vi "CODMn断电保存全局变量.vi"() -> ()   [LabVIEW 2016, in "斯坦道CODMn.lvlib"]
panel:
  in  "远程校准量程":enum16{"L", "H"}(ring)
  in  "远程自动校准浓度":dbl
  in  "CODMn仪器参数":T1 {"单位" items=["ug/L", "mg/L"]}
  out "测量数据区":T2 {"单位" items=["ug/L", "mg/L", "ppm", "mg/m3", "cm", "ppb", "ug/m3", "%", "nmol/mol", "umol/mol", "MPN/L", "MPN/100ml", "ng/m3", "NTU", "无量纲", "ms/cm", "us/cm", "℃", "mV", "万个/L"]}
  in  "运行周期":T3={"运行模式"=enum."维护模式", "质控频次"=enum."关闭", "空白核查时间"=2, "跨度核查时间"=6, "24H周期设置"=[]} {"跨度核查时间" items=["00H", "01H", "02H", "03H", "04H", "05H", "06H", "07H", "08H", "09H", "10H", "11H", "12H", "13H", "14H", "15H", "16H", "17H", "18H", "19H", "20H", "21H", "22H", "23H", "关闭"]; "空白核查时间" items=["00H", "01H", "02H", "03H", "04H", "05H", "06H", "07H", "08H", "09H", "10H", "11H", "12H", "13H", "14H", "15H", "16H", "17H", "18H", "19H", "20H", "21H", "22H", "23H", "关闭"]}
  in  "标样核查量程选择":enum32{"H", "L", "AUTO"}(ring)=enum."AUTO"
  in  "标样浓度":dbl
  in  "零点核查量程选择":enum32{"H", "L", "AUTO"}(ring)=enum."AUTO"
  in  "零点核查浓度":dbl
  in  "MB通信方式选择":enum16{"串口", "TCP"}(ring)
  in  "PORT":string="502"
  in  "IP":string="192.168.1.202"
  in  "Slave ID":u8=1
  in  "Serial Config":T4={"baud rate (bps)"=115200, "stop bits"=10, "parity"=0, "flow control"=0, "timeout"=1000, "retries"=1} {"stop bits" items=["1.0"=10, "1.5"=15, "2.0"=20]; "flow control" items=["None", "XON/XOFF", "RTS/CTS", "XON/XOFF & RTS/CTS", "DTR/DSR", "XON/XOFF & DTR/DSR"]; "parity" items=["None", "Odd", "Even", "Mark", "Space"]}
  in  "Error in":errorcluster
  in  "VISA resource name":refnum<visa-resource-name>="COM4" caption="VISA资源名称"
  in  "常规版/认证版":enum16{"常规版", "认证版", "浮台版"}(ring)
  out "启动时间":timestamp format="%<%Y/%m/%d %H:%M:%S>T"
  in  "高切低阈值:":dbl
  in  "低切高阈值:":dbl
  in  "自动切换量程:":enum16{"关闭", "自动切换测一次", "自动切换测两次"}(ring)
  in  "跨度液浓度":dbl
  in  "CODMn跨度量程选择":enum32{"H", "L", "AUTO"}(ring)=enum."AUTO"
  out "测量模式(公式)":u16(ring) items=["水样测试"=1, "标样核查"=2, "零点核查"=3, "跨度核查"=4, "空白测试"=5, "平行样"=6, "加标回收"=7]
  in  "定时控制":T5
  # "标样浓度："
  # "跨度液浓度："
  # "标样量程选择："
  # "零点核查浓度："
  # "零点量程选择："
  # "MBTCP参数"
  # "mg/L"
  # "运行模式："
  # "质控频次："
  # "空白核查时间："
  # "跨度核查时间："
  # "MB串口参数"
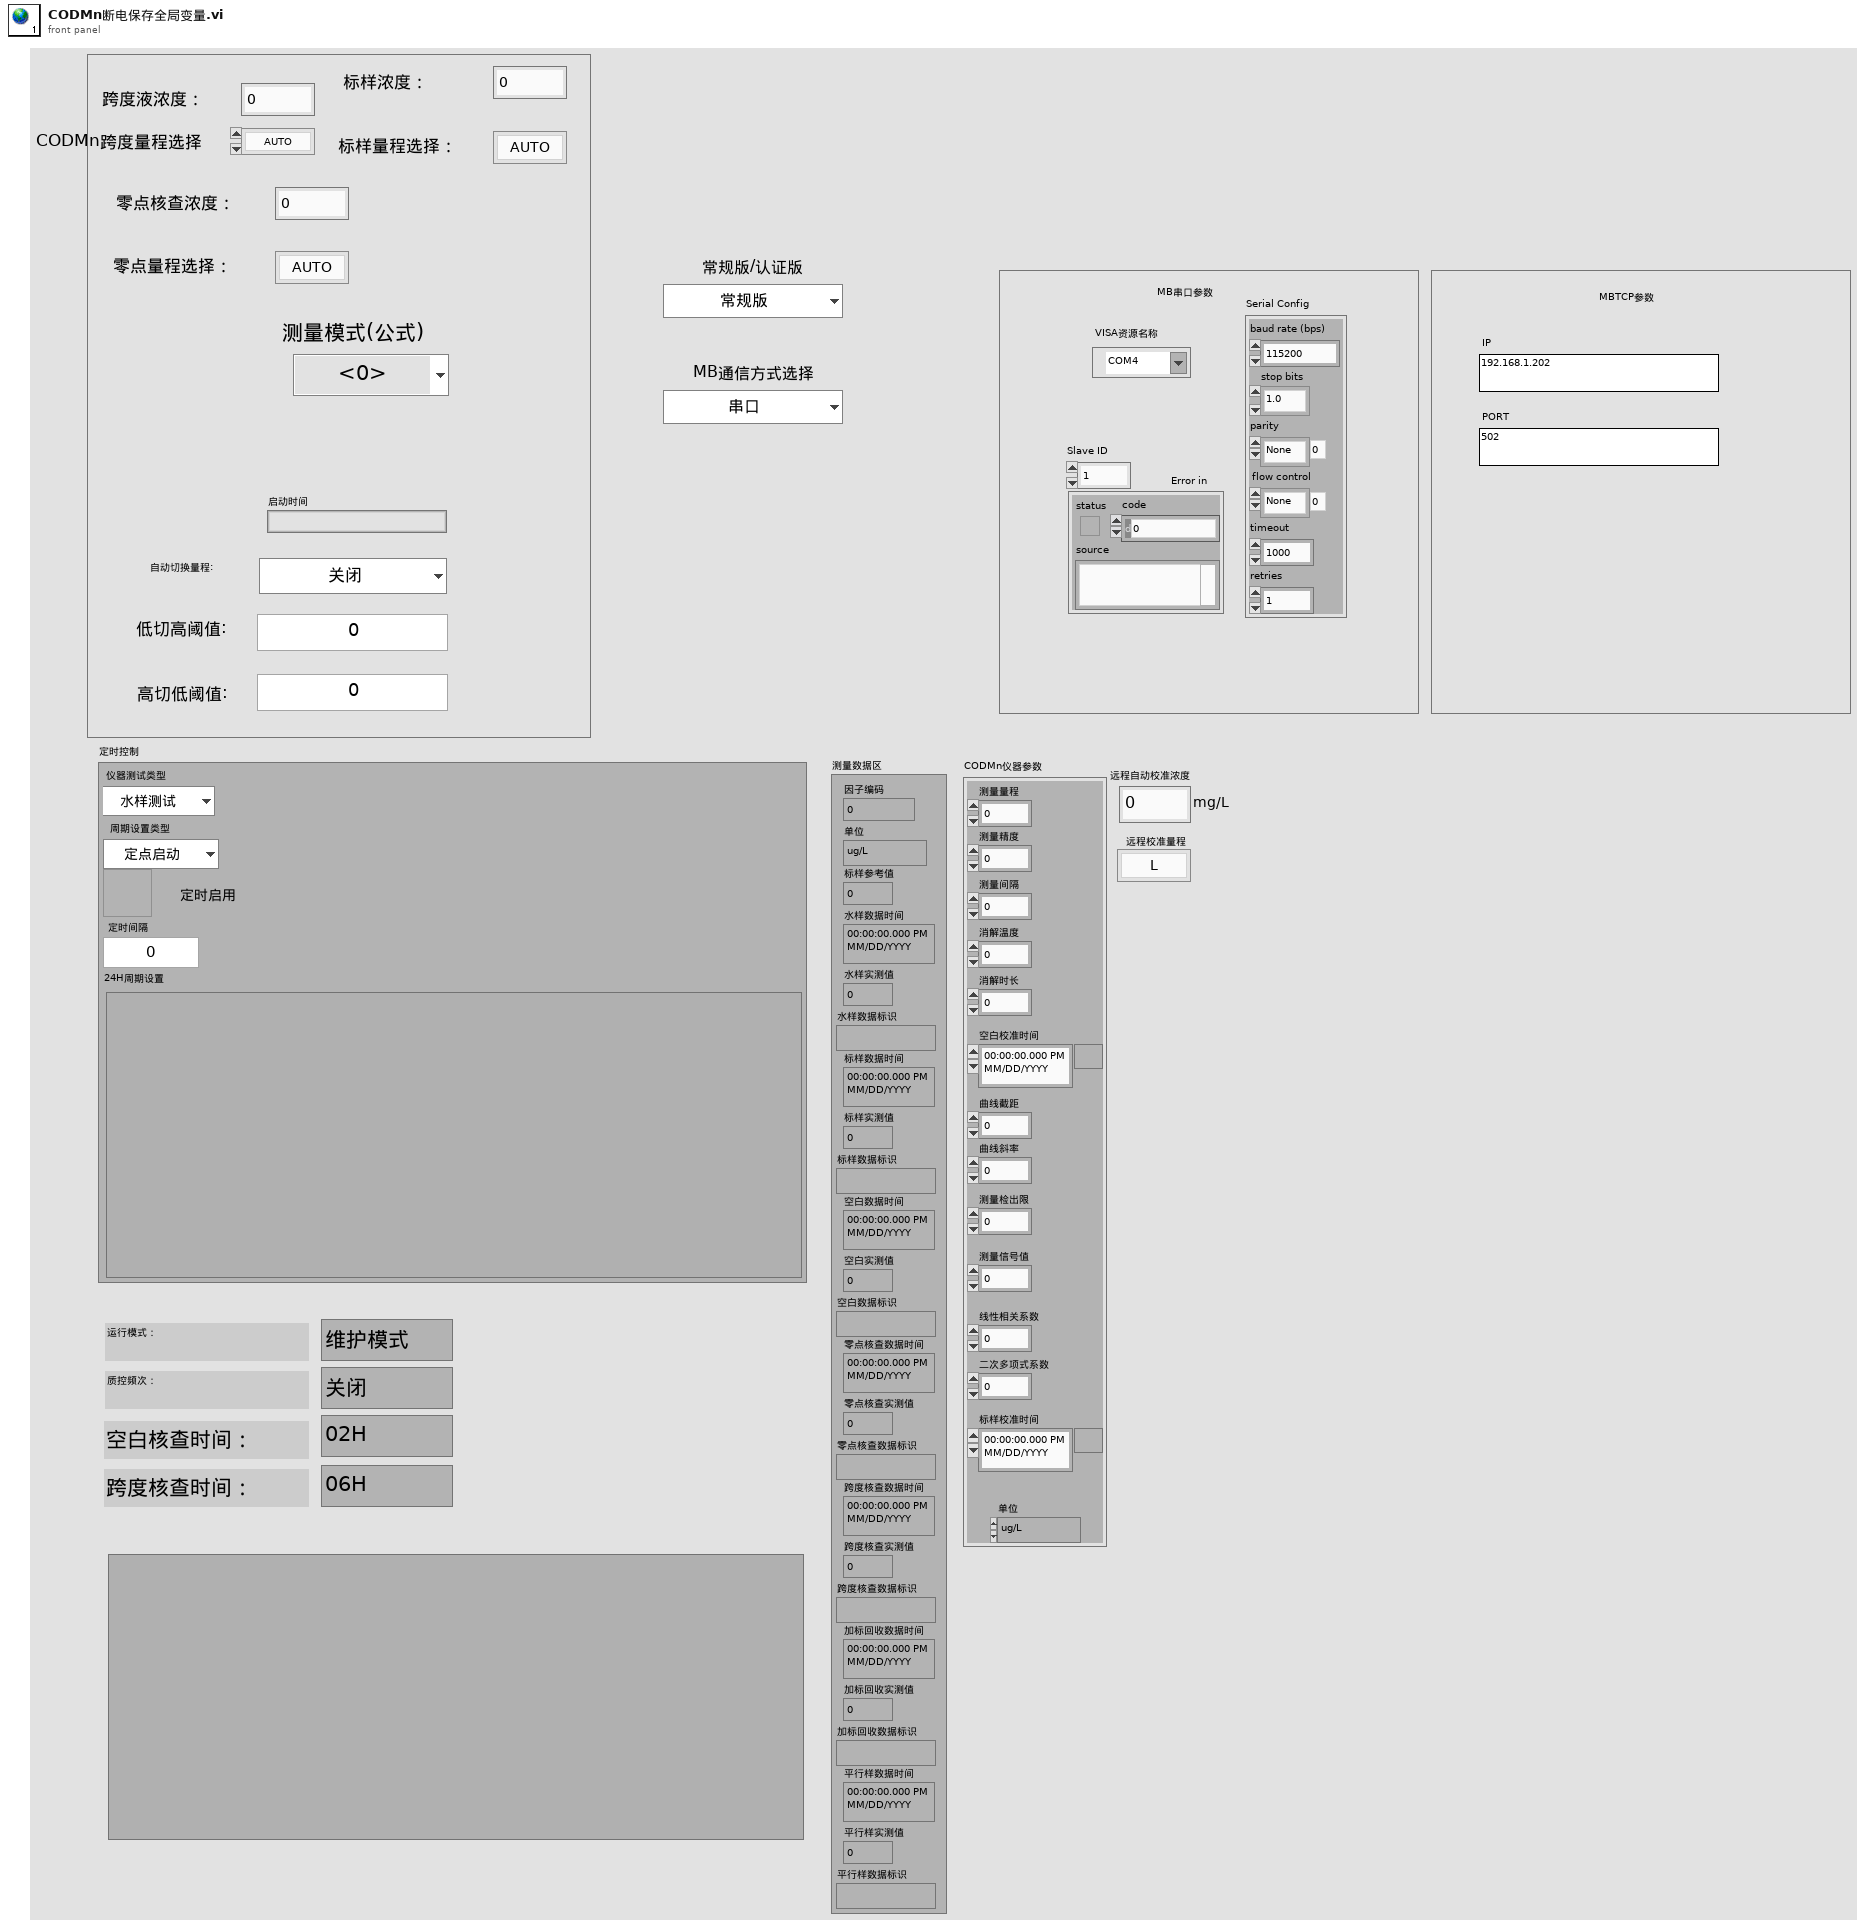
[diagram p1: front panel]
types:
  T1 = cluster{"测量量程":dbl, "测量精度":dbl, "测量间隔":dbl, "消解温度":dbl, "消解时长":dbl, "空白校准时间":timestamp, "曲线截距":dbl, "曲线斜率":dbl, "测量检出限":dbl, "测量信号值":dbl, "线性相关系数":dbl, "二次多项式系数":dbl, "标样校准时间":timestamp, "单位":u16}
  T2 = cluster{"因子编码":u32, "单位":u16, "标样参考值":sgl, "水样数据时间":timestamp, "水样实测值":sgl, "水样数据标识":string, "标样数据时间":timestamp, "标样实测值":sgl, "标样数据标识":string, "空白数据时间":timestamp, "空白实测值":sgl, "空白数据标识":string, "零点核查数据时间":timestamp, "零点核查实测值":sgl, "零点核查数据标识":string, "跨度核查数据时间":timestamp, "跨度核查实测值":sgl, "跨度核查数据标识":string, "加标回收数据时间":timestamp, "加标回收实测值":sgl, "加标回收数据标识":string, "平行样数据时间":timestamp, "平行样实测值":sgl, "平行样数据标识":string}
  T3 = cluster{"运行模式":enum16{"维护模式", "常规模式", "应急模式", "质控模式"}, "质控频次":enum16{"关闭", "每天", "星期一", "星期二", "星期三", "星期四", "星期五", "星期六", "星期日"}, "空白核查时间":u16, "跨度核查时间":u16, "24H周期设置":bool[]}
  T4 = cluster{"baud rate (bps)":u32, "stop bits":u16, "parity":u16, "flow control":u16, "timeout":u32, "retries":i32}
  T5 = cluster{"仪器测试类型":enum16{"水样测试", "零点核查", "标样核查", "空白测试", "跨度核查", "加标回收", "平行样", "校零", "校标"}, "周期设置类型":enum16{"定点启动", "间隔启动"}, "定时功能启用":bool, "定时间隔":dbl, "24H周期设置":bool[]}
diagram:
